vi "Process_HAILO_DataPacket.vi"(8 "error in (no error)":errorcluster, 11 "Data Packet":string) -> (0 "error out":errorcluster, 1 "Sensor Packets Returned":i32, 2 "Sensor Readings (Signed)":i16[](array[numeric]), 3 "Time":u32)   [LabVIEW 2016]
panel:
  out "raw byte array":u8[](array[numeric])
  out "Time Packet":string
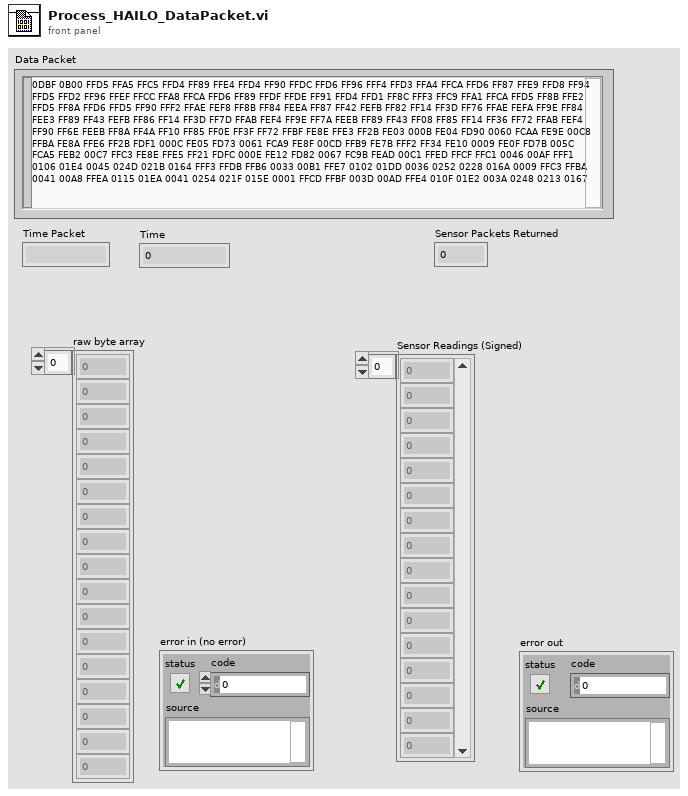
[diagram p1: front panel]
types:
  T1 = enum16{"big-endian, network order", "native, host order", "little-endian"}
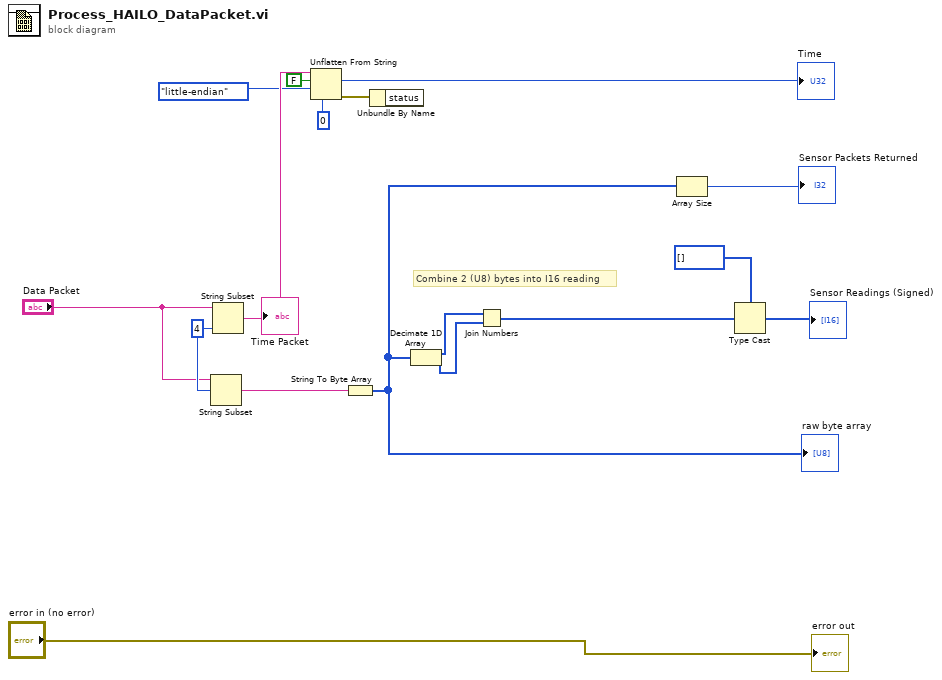
[diagram p0: block diagram]
diagram:
  w17 = 4 ("length (rest)")
  # "Combine 2 (U8) bytes into I16 reading"
  n1 = String Subset(string="Data Packet", offset (0)=w17) -> (substring=w13:string)  [unwired: 1 in]
  n2 = String Subset(string="Data Packet", length (rest)=w17) -> (substring=w16:string)  [unwired: 1 in]
  "Time Packet" <- w16
  n3 = Unflatten From String(type=u32 0 ("default (0 U32)"), binary string=w16, data includes array or string size? (T)=FALSE, byte order (0:big-endian, network order)=T1."little-endian") -> (value=→"Time":u32, error out=w1:errorcluster)  [unwired: 1 in, 1 out]
  n4 = String To Byte Array(string=w13) -> (unsigned byte array=w12:u8[])
  "raw byte array" <- w12
  n5 = Unbundle By Name(w1) -> ()  [unwired: 1 out]
  n6 = Decimate 1D Array(w12) -> (w9:u8[], w8:u8[])
  n7 = Join Numbers(hi=w9, lo=w8) -> ((hi.lo)=w6:u16[])
  n8 = Array Size(array=w12) -> (size(s)=→"Sensor Packets Returned":i32)
  n9 = Type Cast(type=i16[] [], x=w6) -> (*(type *) &x=→"Sensor Readings (Signed)":i16[])
  "error out" <- "error in (no error)"
